vi "Implement IIR Direct Filter for N Specs and N Chan (CDB).vi"(7 "reset Filters":bool[](array[boolean]), 8 "error in (no error)":errorcluster, 9 "Forward Coefficients":dbl[][](array[numeric]) format="%0.2f", 10 "Reverse Coefficients":dbl[][](array[numeric]) format="%0.2f", 11 "arrWaveforms In":waveform(cdb)[](array[waveform])) -> (0 "error out":errorcluster, 3 "arrWaveforms Out":waveform(cdb)[](array[waveform]))   [LabVIEW 2020, in "NI_MAPro.lvlib"]
uses:
  NI_MAPro.lvlib
  NI_MABase.lvlib
  NI_AALBase.lvlib
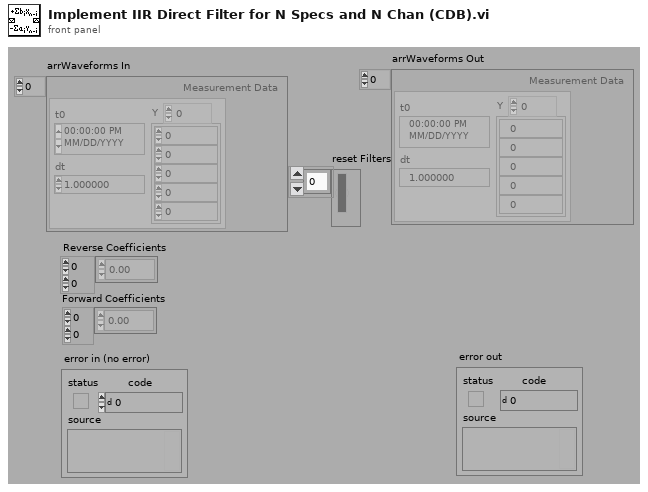
[diagram p1: front panel]
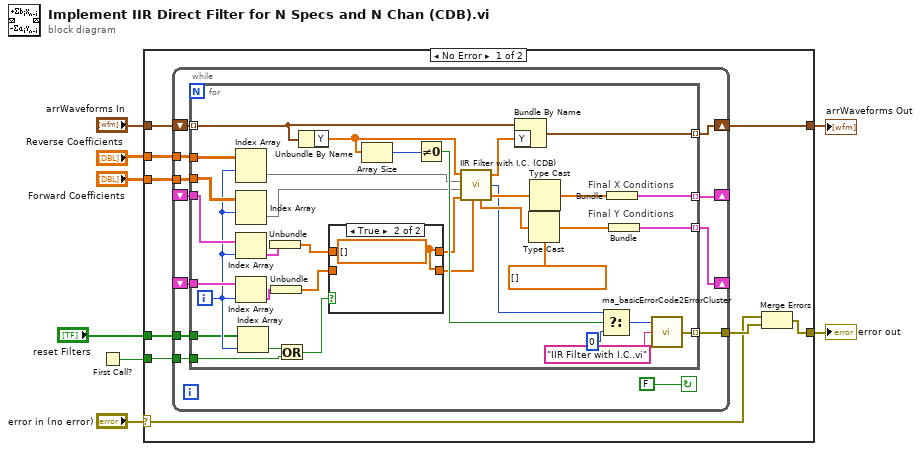
[diagram p0: block diagram]
diagram:
  n1 = First Call?() -> (First Call?: T/F=w2:bool)
  n2 = case shown="No Error" "error in (no error)" {
    selector: "error in (no error)" -> [w14 w69]
    tunnel: [w16 w69] -> w7
    tunnel: "reset Filters" -> [w15 _]
    tunnel: [w13 w68] -> w6
    tunnel: "arrWaveforms In" -> [w12 w68]
    tunnel: "Reverse Coefficients" -> [w11 _]
    tunnel: "Forward Coefficients" -> [w10 _]
    tunnel: w2 -> [w9 _]
    frame No Error {
      n3 = while {
        tunnel: w15 -> [w19]
        tunnel: [w20] -> w17
        tunnel: w11 -> [w22]
        tunnel: w10 -> [w23]
        shift-left: w12 -> [w24]
        shift-right: [w25] -> w13
        shift-left: _ -> [w28]
        shift-right: [w26] -> _
        shift-left: _ -> [w29]
        shift-right: [w27] -> _
        tunnel: w9 -> [w18]
        stop <- FALSE continue-if-true
        n4 = for {
          tunnel: w29 -> [w61]
          tunnel: w28 -> [w62]
          tunnel: [w54] -> w27 mode=indexing
          tunnel: [w57] -> w26 mode=indexing
          tunnel: [w52] -> w25 mode=indexing
          tunnel: w24 -> [w43] mode=indexing
          tunnel: w22 -> [w60]
          tunnel: w23 -> [w59]
          tunnel: [w39] -> w20 mode=indexing
          tunnel: w19 -> [w40]
          tunnel: w18 -> [w31]
          i -> [w41]
          w63 = cdb[] [] ("type for the shift register")
          # "Final Y Conditions"
          # "Final X Conditions"
          n5 = Index Array(array=w60, index (row)=w41) -> (element=w51:dbl[])  [unwired: 1 in]
          n6 = Index Array(array=w59, index (row)=w41) -> (element=w50:dbl[])  [unwired: 1 in]
          n7 = Index Array(array=w61, index=w41) -> (element=w53:cluster{"type for the shift register":cdb[]})
          n8 = Index Array(array=w62, index=w41) -> (element=w56:cluster{"type for the shift register":cdb[]})
          n9 = Index Array(array=w40, index=w41) -> (element=w32:bool)
          n10 = Unbundle(w53) -> ("type for the shift register"=w45:cdb[])
          n11 = Unbundle(w56) -> ("type for the shift register"=w46:cdb[])
          n12 = Or(x=w32, y=w31) -> (x .or. y?=w30:bool)
          n13 = Unbundle By Name(w43) -> ("Y"=w33:cdb[])
          n14 = case shown="True" w30 {
            tunnel: w46 -> [w66 _]
            tunnel: [w66 w67] -> w47
            tunnel: w45 -> [w65 _]
            tunnel: [w65 w67] -> w44
            frame False {
            }
            frame True {
              w67 = cdb[] [] ("type for the shift register")
            }
          }
          n15 = Array Size(array=w33) -> (size(s)=w34:i32)
          n16 = Not Equal To 0?(x=w34) -> (x != 0?=w64:bool)
          n17 = call "IIR Filter with I.C. (CDB).vi"("Initial Y Conditions"=w47, "Initial X Conditions"=w44, "Forward Coefficients"=w50, "Reverse Coefficients"=w51, "X"=w33) -> ("Final X Conditions"=w48:cdb[], "Final Y Conditions"=w49:cdb[], "error"=w35:i32, "Filtered X"=w42:cdb[])  [unwired: 2 in]
          n18 = Bundle By Name(cluster=w43, "Y"=w42) -> (w52:waveform(cdb))
          n19 = Type Cast(type=w63, x=w49) -> (*(type *) &x=w58:cdb[])
          n20 = Type Cast(type=w63, x=w48) -> (*(type *) &x=w55:cdb[])
          n21 = Select(t=w35, s=w64, f=0) -> (s? t:f=w36:i32)
          n22 = Bundle("type for the shift register"=w55) -> (w54:cluster{"type for the shift register":cdb[]})  [unwired: 1 in]
          n23 = Bundle("type for the shift register"=w58) -> (w57:cluster{"type for the shift register":cdb[]})  [unwired: 1 in]
          n24 = call "ma_basicErrorCode2ErrorCluster.vi"("subVI name"="IIR Filter with I.C..vi", "Error Code"=w36) -> ("error out"=w39:errorcluster)  [unwired: 1 in]
        }
      }
      n25 = Merge Errors(w14, w17) -> (w16:errorcluster)
    }
    frame Error {
    }
  }
  "error out" <- w7
  "arrWaveforms Out" <- w6
